vi "DEMO_04_CONFIG.vi"() -> ()   [LabVIEW 2014]
uses:
  <vilib>/Instr/_visa.llb/VISA Configure Serial Port (Instr).vi
panel:
  out "最小电压 3":dbl
  out "最小电压 2":dbl
  out "最大电压 3":dbl
  out "最大电压 2":dbl
  in  "奇偶":enum16{"None", "Odd", "Even", "Mark", "Space"}(ring) caption="校验"
  in  "波特率":u32(ring)=9600 items=["75"=75, "110"=110, "134"=134, "150"=150, "300"=300, "600"=600, "1200"=1200, "1800"=1800, "2400"=2400, "4800"=4800, "7200"=7200, "9600"=9600, "14400"=14400, "19200"=19200, "28800"=28800, "38400"=38400, "56000"=56000, "57600"=57600, "115200"=115200, "128000"=128000, "230400"=230400]
  in  "VISA资源名称":refnum<visa-resource-name>="COM1"
  out "三路负载":dbl
  out "二路负载":dbl
  out "一路负载":dbl
  out "最小位移":dbl
  out "三路功率":dbl
  out "二路功率":dbl
  out "一路功率":dbl
  out "三路最大位移":dbl
  out "二路最大位移":dbl
  out "一路最大位移":dbl
  out "最大电压":dbl
  out "最小电压":dbl
  in  "读系统参数":bool
  in  "上位机控制":bool
  in  "打开串口":bool
  # "哈尔滨芯明天科技有限公司例程: 读取系统设置"
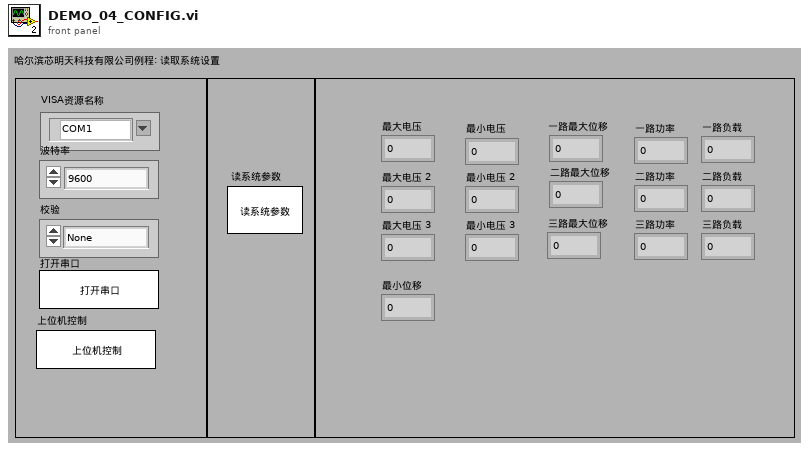
[diagram p1: front panel]
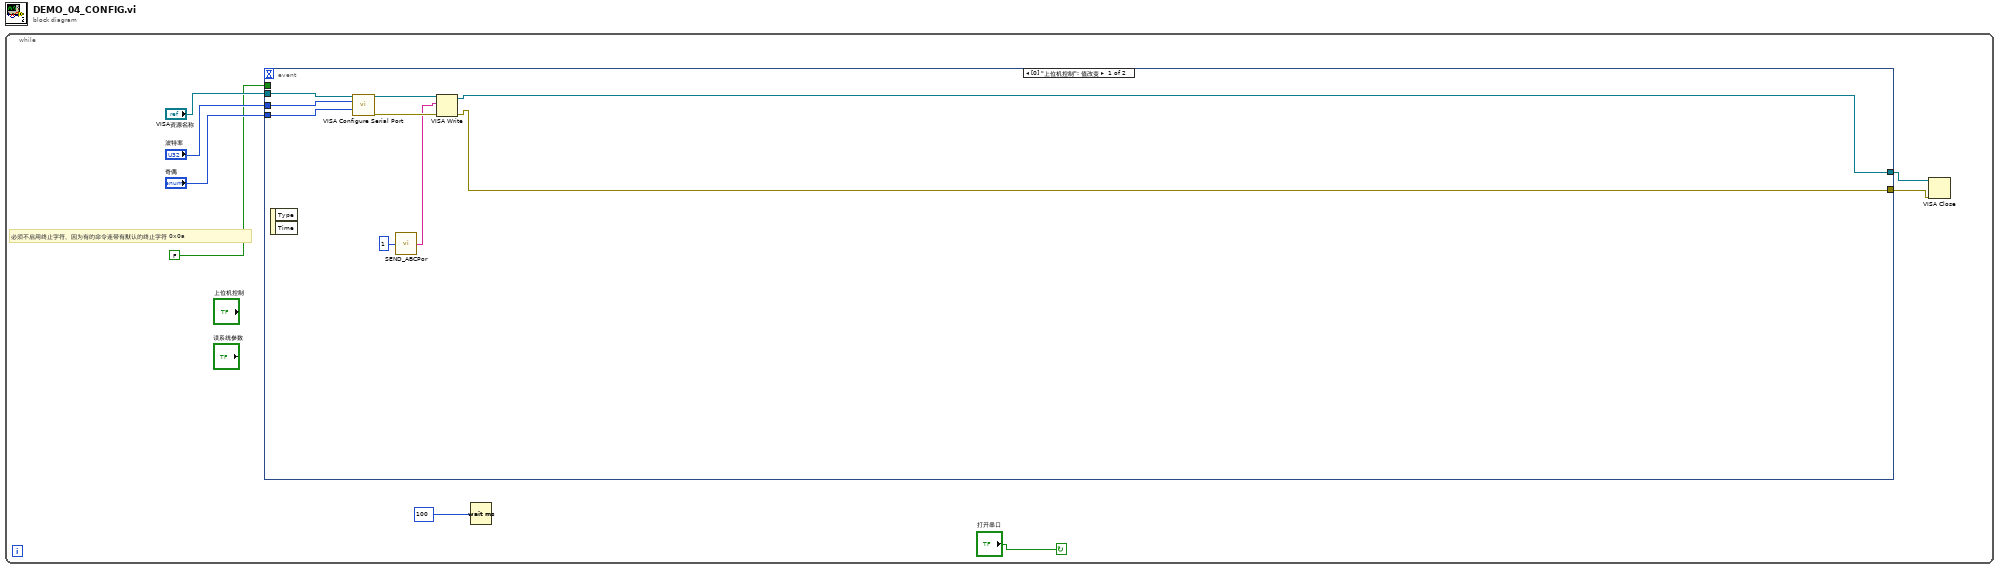
[diagram p0: block diagram]
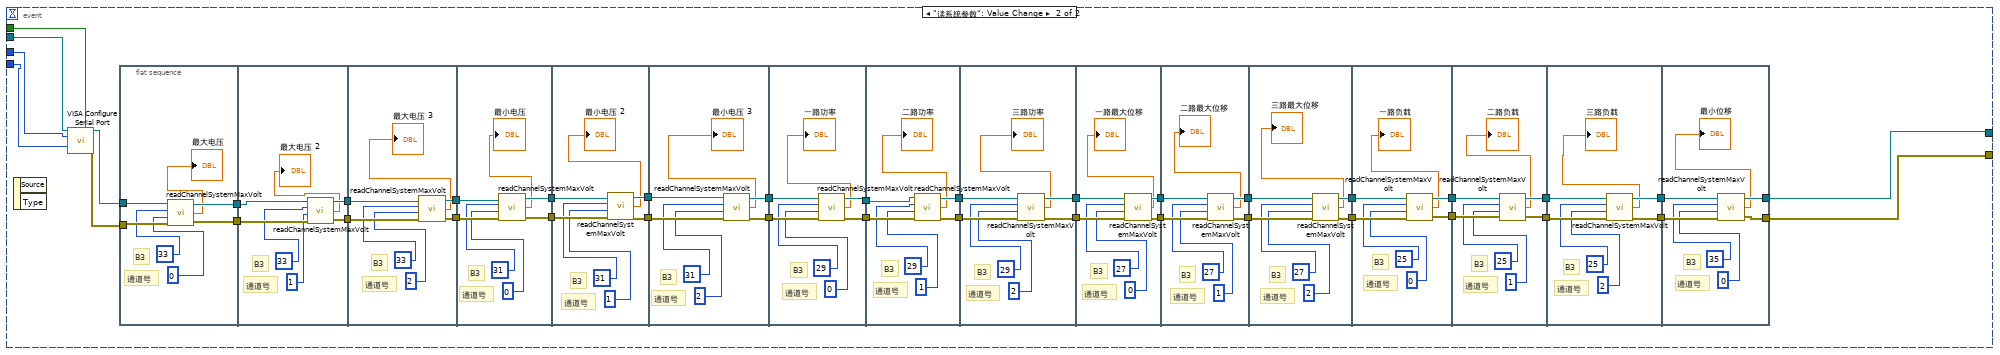
[diagram p2: hidden frame]
diagram:
  n1 = while {
    stop <- "打开串口" continue-if-true
    # "必须不启用终止字符、因为有的命令连带有默认的终止字符 0x0a"
    n2 = event shown="[0] \"上位机控制\": 值改变" {
      selector: _ -> [_ _]
      dyn-events: _ -> [_ _]
      timeout: _ -> [_ _]
      tunnel: "VISA资源名称" -> [w17 w53]
      tunnel: "波特率" -> [w16 w54]
      tunnel: "奇偶" -> [w15 w55]
      tunnel: [w12 w20] -> w3
      tunnel: [w11 w19] -> w2
      tunnel: FALSE -> [_ w18]
      event "上位机控制": Value Change {
        n3 = event-data() -> ()  [unwired: 1 in, 2 out]
        n4 = call-poly "VISA Configure Serial Port"("VISA resource name"=w17, "baud rate (9600)"=w16, "parity (0:none)"=w15) -> ("VISA resource name out"=w13:refnum<visa-resource-name>, "error out"=w14:errorcluster)  [unwired: 11 in]
        n5 = call "SEND_ABCPor.vi"("设备地址 1 开始"=1) -> ("输出字符串"=w9:string)
        n6 = VISA Write(VISA resource name=w13, write buffer=w9, error in (no error)=w14) -> (VISA resource name out=w12:refnum<visa-resource-name>, error out=w11:errorcluster)  [unwired: 1 out]
      }
      event "读系统参数": Value Change {
        n7 = event-data() -> ()  [unwired: 1 in, 2 out]
        n8 = call-poly "VISA Configure Serial Port"("VISA resource name"=w53, "Enable Termination\nChar (T)"=w18, "baud rate (9600)"=w54, "parity (0:none)"=w55) -> ("VISA resource name out"=w52:refnum<visa-resource-name>, "error out"=w51:errorcluster)  [unwired: 10 in]
        n9 = flat-sequence {
          tunnel: w52 -> [w62]
          tunnel: w51 -> [w61]
          tunnel: [w58] -> w50
          tunnel: [w57] -> w21
          tunnel: w50 -> [w69]
          tunnel: [w68] -> w49
          tunnel: [w67] -> w22
          tunnel: w21 -> [w66]
          tunnel: w49 -> [w76]
          tunnel: [w75] -> w48
          tunnel: [w74] -> w23
          tunnel: w22 -> [w73]
          tunnel: w48 -> [w83]
          tunnel: [w82] -> w47
          tunnel: [w81] -> w24
          tunnel: w23 -> [w80]
          tunnel: w47 -> [w90]
          tunnel: [w89] -> w46
          tunnel: [w88] -> w25
          tunnel: w24 -> [w87]
          tunnel: w46 -> [w97]
          tunnel: [w96] -> w45
          tunnel: [w95] -> w26
          tunnel: w25 -> [w94]
          tunnel: w45 -> [w104]
          tunnel: [w103] -> w44
          tunnel: [w102] -> w27
          tunnel: w26 -> [w101]
          tunnel: w44 -> [w111]
          tunnel: [w110] -> w43
          tunnel: [w109] -> w28
          tunnel: w27 -> [w108]
          tunnel: w43 -> [w118]
          tunnel: [w117] -> w42
          tunnel: [w116] -> w29
          tunnel: w28 -> [w115]
          tunnel: w42 -> [w125]
          tunnel: [w124] -> w41
          tunnel: [w123] -> w30
          tunnel: w29 -> [w122]
          tunnel: w41 -> [w132]
          tunnel: [w131] -> w40
          tunnel: [w130] -> w31
          tunnel: w30 -> [w129]
          tunnel: w40 -> [w139]
          tunnel: [w138] -> w39
          tunnel: [w137] -> w32
          tunnel: w31 -> [w136]
          tunnel: w39 -> [w146]
          tunnel: [w145] -> w38
          tunnel: [w144] -> w33
          tunnel: w32 -> [w143]
          tunnel: w38 -> [w153]
          tunnel: [w152] -> w37
          tunnel: [w151] -> w34
          tunnel: w33 -> [w150]
          tunnel: w37 -> [w160]
          tunnel: [w159] -> w36
          tunnel: [w158] -> w35
          tunnel: w34 -> [w157]
          tunnel: w36 -> [w167]
          tunnel: [w166] -> w20
          tunnel: [w165] -> w19
          tunnel: w35 -> [w164]
          frame #0 {
            # "通道号"
            # "B3"
            n10 = call "readChannelSystemMaxVolt.vi"("error out 2"=w61, "通道号"=0 ("B3"), "B3"=33, "VISA resource name out 2"=w62) -> ("error out"=w57:errorcluster, "输出变量"=→"最大电压":dbl, "VISA resource name out"=w58:refnum<visa-resource-name>)
          }
          frame #1 {
            # "通道号"
            # "B3"
            n11 = call "readChannelSystemMaxVolt.vi"("error out 2"=w66, "通道号"=1 ("B3"), "B3"=33, "VISA resource name out 2"=w69) -> ("error out"=w67:errorcluster, "输出变量"=→"最大电压 2":dbl, "VISA resource name out"=w68:refnum<visa-resource-name>)
          }
          frame #2 {
            # "通道号"
            # "B3"
            n12 = call "readChannelSystemMaxVolt.vi"("error out 2"=w73, "通道号"=2 ("B3"), "B3"=33, "VISA resource name out 2"=w76) -> ("error out"=w74:errorcluster, "输出变量"=→"最大电压 3":dbl, "VISA resource name out"=w75:refnum<visa-resource-name>)
          }
          frame #3 {
            # "通道号"
            # "B3"
            n13 = call "readChannelSystemMaxVolt.vi"("error out 2"=w80, "通道号"=0 ("B3"), "B3"=31, "VISA resource name out 2"=w83) -> ("error out"=w81:errorcluster, "输出变量"=→"最小电压":dbl, "VISA resource name out"=w82:refnum<visa-resource-name>)
          }
          frame #4 {
            # "通道号"
            # "B3"
            n14 = call "readChannelSystemMaxVolt.vi"("error out 2"=w87, "通道号"=1 ("B3"), "B3"=31, "VISA resource name out 2"=w90) -> ("error out"=w88:errorcluster, "输出变量"=→"最小电压 2":dbl, "VISA resource name out"=w89:refnum<visa-resource-name>)
          }
          frame #5 {
            # "通道号"
            # "B3"
            n15 = call "readChannelSystemMaxVolt.vi"("error out 2"=w94, "通道号"=2 ("B3"), "B3"=31, "VISA resource name out 2"=w97) -> ("error out"=w95:errorcluster, "输出变量"=→"最小电压 3":dbl, "VISA resource name out"=w96:refnum<visa-resource-name>)
          }
          frame #6 {
            # "通道号"
            # "B3"
            n16 = call "readChannelSystemMaxVolt.vi"("error out 2"=w101, "通道号"=0 ("B3"), "B3"=29, "VISA resource name out 2"=w104) -> ("error out"=w102:errorcluster, "输出变量"=→"一路功率":dbl, "VISA resource name out"=w103:refnum<visa-resource-name>)
          }
          frame #7 {
            # "通道号"
            # "B3"
            n17 = call "readChannelSystemMaxVolt.vi"("error out 2"=w108, "通道号"=1 ("B3"), "B3"=29, "VISA resource name out 2"=w111) -> ("error out"=w109:errorcluster, "输出变量"=→"二路功率":dbl, "VISA resource name out"=w110:refnum<visa-resource-name>)
          }
          frame #8 {
            # "通道号"
            # "B3"
            n18 = call "readChannelSystemMaxVolt.vi"("error out 2"=w115, "通道号"=2 ("B3"), "B3"=29, "VISA resource name out 2"=w118) -> ("error out"=w116:errorcluster, "输出变量"=→"三路功率":dbl, "VISA resource name out"=w117:refnum<visa-resource-name>)
          }
          frame #9 {
            # "通道号"
            # "B3"
            n19 = call "readChannelSystemMaxVolt.vi"("error out 2"=w122, "通道号"=0 ("B3"), "B3"=27, "VISA resource name out 2"=w125) -> ("error out"=w123:errorcluster, "输出变量"=→"一路最大位移":dbl, "VISA resource name out"=w124:refnum<visa-resource-name>)
          }
          frame #10 {
            # "通道号"
            # "B3"
            n20 = call "readChannelSystemMaxVolt.vi"("error out 2"=w129, "通道号"=1 ("B3"), "B3"=27, "VISA resource name out 2"=w132) -> ("error out"=w130:errorcluster, "输出变量"=→"二路最大位移":dbl, "VISA resource name out"=w131:refnum<visa-resource-name>)
          }
          frame #11 {
            # "通道号"
            # "B3"
            n21 = call "readChannelSystemMaxVolt.vi"("error out 2"=w136, "通道号"=2 ("B3"), "B3"=27, "VISA resource name out 2"=w139) -> ("error out"=w137:errorcluster, "输出变量"=→"三路最大位移":dbl, "VISA resource name out"=w138:refnum<visa-resource-name>)
          }
          frame #12 {
            # "通道号"
            # "B3"
            n22 = call "readChannelSystemMaxVolt.vi"("error out 2"=w143, "通道号"=0 ("B3"), "B3"=25, "VISA resource name out 2"=w146) -> ("error out"=w144:errorcluster, "输出变量"=→"一路负载":dbl, "VISA resource name out"=w145:refnum<visa-resource-name>)
          }
          frame #13 {
            # "通道号"
            # "B3"
            n23 = call "readChannelSystemMaxVolt.vi"("error out 2"=w150, "通道号"=1 ("B3"), "B3"=25, "VISA resource name out 2"=w153) -> ("error out"=w151:errorcluster, "输出变量"=→"二路负载":dbl, "VISA resource name out"=w152:refnum<visa-resource-name>)
          }
          frame #14 {
            # "通道号"
            # "B3"
            n24 = call "readChannelSystemMaxVolt.vi"("error out 2"=w157, "通道号"=2 ("B3"), "B3"=25, "VISA resource name out 2"=w160) -> ("error out"=w158:errorcluster, "输出变量"=→"三路负载":dbl, "VISA resource name out"=w159:refnum<visa-resource-name>)
          }
          frame #15 {
            # "通道号"
            # "B3"
            n25 = call "readChannelSystemMaxVolt.vi"("error out 2"=w164, "通道号"=0 ("B3"), "B3"=35, "VISA resource name out 2"=w167) -> ("error out"=w165:errorcluster, "输出变量"=→"最小位移":dbl, "VISA resource name out"=w166:refnum<visa-resource-name>)
          }
        }
      }
    }
    n26 = Wait (ms)(milliseconds to wait=100) -> ()  [unwired: 1 out]
    n27 = VISA Close(VISA resource name=w3, error in (no error)=w2) -> ()  [unwired: 1 out]
  }
